vi "Door Access System.vi"() -> ()   [LabVIEW 2019]
panel:
  out "3":i32
  out "2":i32
  out "1":i32
  out "Wrong":bool
  out "Correct":bool
  out "0":i32
  in  "D":bool
  in  "C":bool
  in  "B":bool
  in  "A":bool
  in  "E":bool
  in  "F":bool
  in  "9":bool
  in  "8":bool
  in  "7":bool
  in  "6":bool
  in  "5":bool
  in  "4":bool
  in  "3":bool
  in  "2":bool
  in  "1":bool
  in  "0":bool
  out "Keypad Value":i32[](array[numeric])
  in  "stop 3":bool
  in  "stop 2":bool
  out "7-segment":T1
  in  "stop":bool
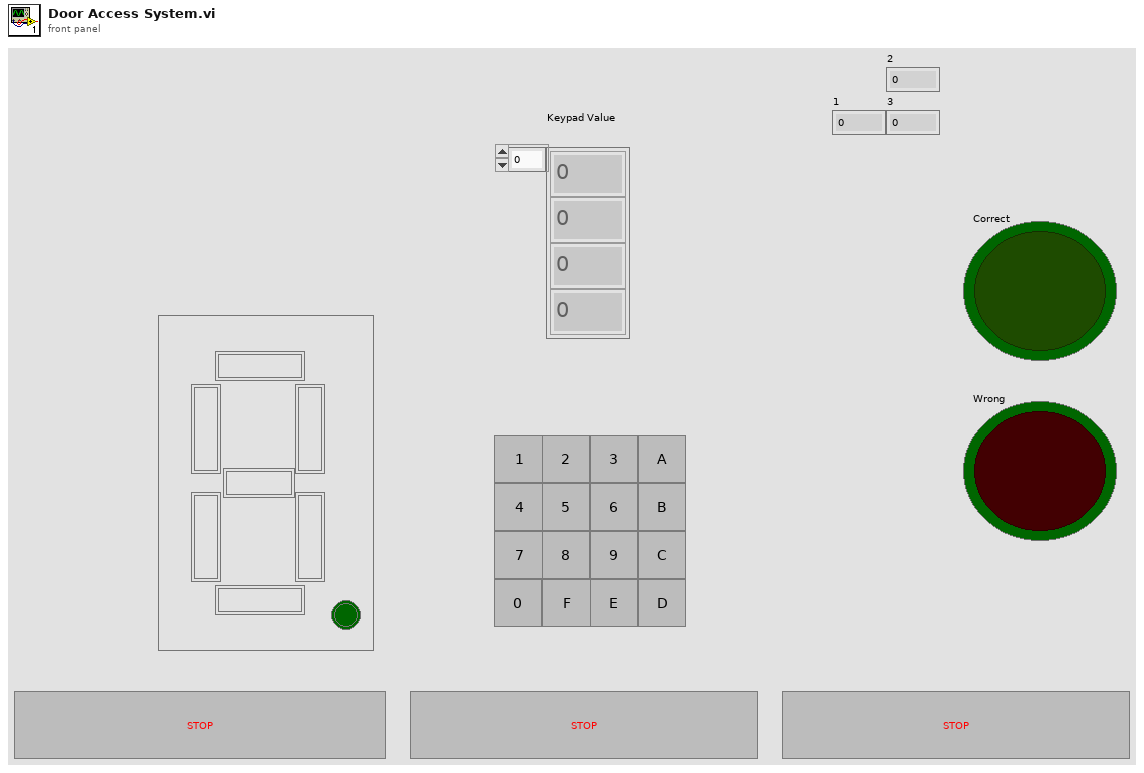
[diagram p1: front panel]
types:
  T1 = cluster{"a":bool, "b":bool, "c":bool, "d":bool, "e":bool, "f":bool, "g":bool, "DP":bool}
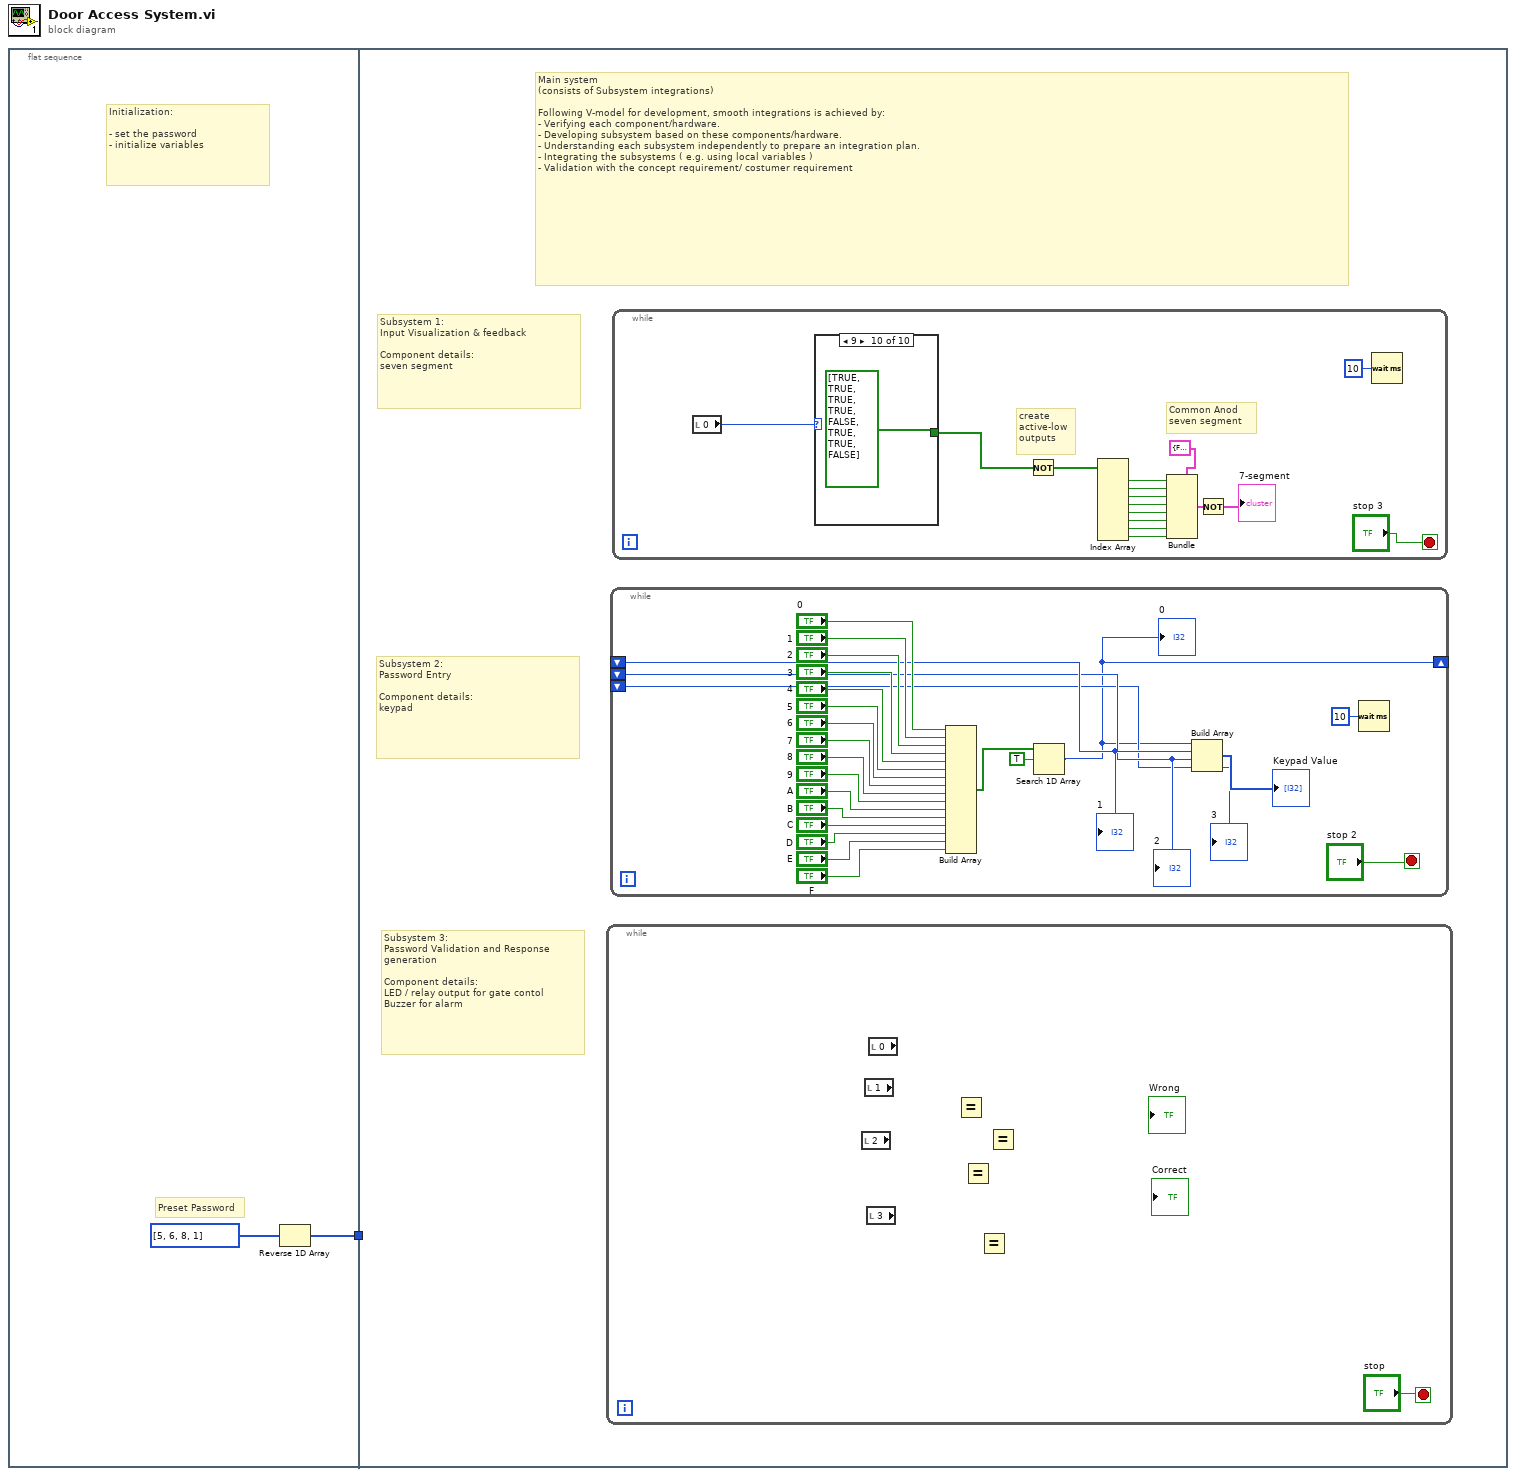
[diagram p0: block diagram]
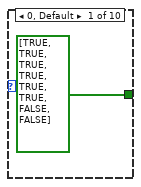
[diagram p2: hidden frame]
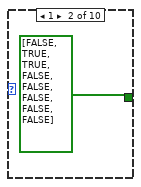
[diagram p3: hidden frame]
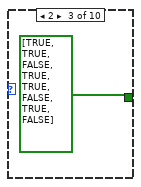
[diagram p4: hidden frame]
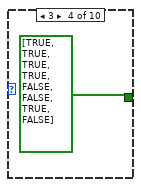
[diagram p5: hidden frame]
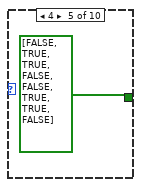
[diagram p6: hidden frame]
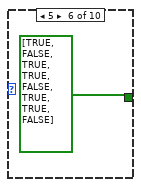
[diagram p7: hidden frame]
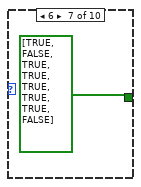
[diagram p8: hidden frame]
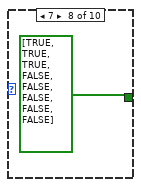
[diagram p9: hidden frame]
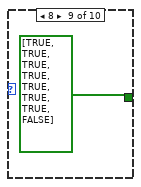
[diagram p10: hidden frame]
diagram:
  n1 = flat-sequence {
    tunnel: [w2] -> w1
    tunnel: w1 -> [_]
    frame #0 {
      # "Preset Password"
      # "Initialization:\n\n- set the password\n- initialize variables"
      n2 = Reverse 1D Array(array=i32[] [5, 6, 8, 1] ("Saved Password")) -> (reversed array=w2:i32[])
    }
    frame #1 {
      # "Subsystem 3:\nPassword Validation and Response generation\n\nComponent details:\nLED / relay output for gate contol\nBuzzer for alarm"
      # "Subsystem 1:\nInput Visualization & feedback\n\nComponent details:\nseven segment"
      # "Main system \n(consists of Subsystem integrations)\n\nFollowing V-model for development, smooth integrations is achieved by:\n- Verifying each component/hardware.\n- Developing subsystem based on these components/hardware.\n- Understanding each subsystem independently to prepare an integration plan.\n- Integrating the subsystems ( e.g. using local variables )\n- Validation with the concept requirement/ costumer requirement"
      # "Subsystem 2:\nPassword Entry\n\nComponent details:\nkeypad"
      n3 = while {
        stop <- "stop" stop-if-true
        n4 = local read "2"() -> ()  [unwired: 1 out]
        n5 = local read "1"() -> ()  [unwired: 1 out]
        n6 = local read "3"() -> ()  [unwired: 1 out]
        n7 = local read "0"() -> ()  [unwired: 1 out]
        n8 = Equal?() -> ()  [unwired: 2 in, 1 out]
        n9 = Equal?() -> ()  [unwired: 2 in, 1 out]
        n10 = Equal?() -> ()  [unwired: 2 in, 1 out]
        n11 = Equal?() -> ()  [unwired: 2 in, 1 out]
      }
      n12 = while {
        shift-right: [w30] -> _
        shift-left: _ -> [w34]
        shift-left: _ -> [w33]
        shift-left: _ -> [w31]
        stop <- "stop 2" stop-if-true
        n13 = Build Array("0", "1", "2", "3", "4", "5", "6", "7", "8", "9", "A", "B", "C", "D", "E", "F") -> (w41:bool[])
        n14 = Search 1D Array(1D array=w41, element=TRUE) -> (index of element=w30:i32)  [unwired: 1 in]
        "0" <- w30
        n15 = Build Array(w30, w34, w33, w31) -> (→"Keypad Value":i32[])
        n16 = Wait (ms)(milliseconds to wait=u32 10) -> ()  [unwired: 1 out]
        "1" <- w34
        "2" <- w33
        "3" <- w31
      }
      n17 = while {
        stop <- "stop 3" stop-if-true
        # "Common Anod \nseven segment"
        # "create\nactive-low\noutputs"
        n18 = local read "0"() -> (w4:i32)
        n19 = case shown="9" w4 {
          tunnel: [bool[] [TRUE, TRUE, TRUE, TRUE, TRUE, TRUE, FALSE, FALSE] ("LED segments 2") bool[] [FALSE, TRUE, TRUE, FALSE, FALSE, FALSE, FALSE, FALSE] ("LED segments 2") bool[] [TRUE, TRUE, FALSE, TRUE, TRUE, FALSE, TRUE, FALSE] ("LED segments 2") bool[] [TRUE, TRUE, TRUE, TRUE, FALSE, FALSE, TRUE, FALSE] ("LED segments 2") bool[] [FALSE, TRUE, TRUE, FALSE, FALSE, TRUE, TRUE, FALSE] ("LED segments 2") bool[] [TRUE, FALSE, TRUE, TRUE, FALSE, TRUE, TRUE, FALSE] ("LED segments 2") bool[] [TRUE, FALSE, TRUE, TRUE, TRUE, TRUE, TRUE, FALSE] ("LED segments 2") bool[] [TRUE, TRUE, TRUE, FALSE, FALSE, FALSE, FALSE, FALSE] ("LED segments 2") bool[] [TRUE, TRUE, TRUE, TRUE, TRUE, TRUE, TRUE, FALSE] ("LED segments 2") bool[] [TRUE, TRUE, TRUE, TRUE, FALSE, TRUE, TRUE, FALSE] ("LED segments 2")] -> w18
          frame 0, Default {
          }
          frame 1 {
          }
          frame 2 {
          }
          frame 3 {
          }
          frame 4 {
          }
          frame 5 {
          }
          frame 6 {
          }
          frame 7 {
          }
          frame 8 {
          }
          frame 9 {
          }
        }
        n20 = Not(x=w18) -> (.not. x?=w19:bool[])
        n21 = Index Array "Index Array"(array=w19) -> (element #1=w17:bool, element #2=w16:bool, element #3=w15:bool, element #4=w14:bool, element #5=w13:bool, element #6=w12:bool, element #7=w11:bool, element #8=w10:bool)  [unwired: 8 in]
        n22 = Bundle(cluster=T1 {"a"=FALSE, "b"=FALSE, "c"=FALSE, "d"=FALSE, "e"=FALSE, "f"=FALSE, "g"=FALSE, "DP"=FALSE} ("7-segment"), "a"=w17, "b"=w16, "c"=w15, "d"=w14, "e"=w13, "f"=w12, "g"=w11, "DP"=w10) -> (w8:T1)
        n23 = Not(x=w8) -> (.not. x?=→"7-segment":T1)
        n24 = Wait (ms)(milliseconds to wait=u32 10) -> ()  [unwired: 1 out]
      }
    }
  }
